vi "RampVoltagewithDDSv8.vi"() -> ()   [LabVIEW 2016]
uses:
  <vilib>/DAQmx/write.llb/DAQmx Write (Digital 1D Wfm NChan NSamp).vi
  <vilib>/DAQmx/write.llb/DAQmx Write (Analog 2D DBL NChan NSamp).vi
  <vilib>/DAQmx/create/channels.llb/DAQmx Create Channel (AO-Voltage-Basic).vi
  <vilib>/DAQmx/create/channels.llb/DAQmx Create Channel (DO-Digital Output).vi
  <vilib>/DAQmx/configure/timing.llb/DAQmx Timing (Sample Clock).vi
  <vilib>/DAQmx/configure/trigger.llb/DAQmx Start Trigger (Digital Edge).vi
  <vilib>/DAQmx/miscellaneous.llb/DAQmx Fill In Error Info.vi
  <vilib>/Waveform/DWDTOps.llb/DWDT Boolean Array to Digital.vi
  <vilib>/Waveform/DWDTOps.llb/DWDT Uncompress Digital.vi
  <vilib>/Waveform/DTblOps.llb/DTbl Digital to Analog.vi
  <resource>/objmgr/daqmx.rc
panel:
  in  "Reset P0.1":bool
  in  "Reset P0.0":bool
  in  "DDS Trigger delay (ms)":dbl step=0.01
  in  "DDS Trigger (Port 0 Line 1)":tag="Dev2/port0/line1"
  out "Digital Output":cluster{i32, dbl, dbl[][]}(graph)={0, 1e-05, [[5.0, 5.0, 5.0, 5.0, 5.0, 5.0, 5.0, 5.0, 5.0, 5.0, 5.0, 5.0, 5.0, 5.0, 5.0, 5.0, 5.0, 5.0, 5.0, 5.0, 5.0, 5.0, 5.0, 5.0, 5.0, 5.0, 5.0, 5.0, 5.0, 5.0, 5.0, 5.0, 5.0, 5.0, 5.0, 5.0, 5.0, 5.0, 5.0, 5.0, 5.0, 5.0, 5.0, 5.0, 5.0, 5.0, 5.0, 5.0, 5.0, 5.0, 5.0, 5.0, 5.0, 5.0, 5.0, 5.0, 5.0, 5.0, 5.0, 5.0, 5.0, 5.0, 5.0, 5.0, 5.0, 5.0, 5.0, 5.0, 5.0, 5.0, 5.0, 5.0, 5.0, 5.0, 5.0, 5.0, 5.0, 5.0, 5.0, 5.0, 5.0, 5.0, 5.0, 5.0, 5.0, 5.0, 5.0, 5.0, 5.0, 5.0, 5.0, 5.0, 5.0, 5.0, 5.0, 5.0, 5.0, 5.0, 5.0, 5.0, 0.0, 0.0, 0.0, 0.0, 0.0, 0.0, 0.0, 0.0, 0.0, 0.0, 0.0, 0.0, 0.0, 0.0, 0.0, 0.0, 0.0, 0.0, 0.0, 0.0, 0.0, 0.0, 0.0, 0.0, 0.0, 0.0, 0.0, 0.0, 0.0, 0.0, 0.0, 0.0, 0.0, 0.0, 0.0, 0.0, 0.0, 0.0, 0.0, 0.0, 0.0, 0.0, 0.0, 0.0, 0.0, 0.0, 0.0, 0.0, 0.0, 0.0, 0.0, 0.0, 0.0, 0.0, 0.0, 0.0, 0.0, 0.0, 0.0, 0.0, 0.0, 0.0, 0.0, 0.0, 0.0, 0.0, 0.0, 0.0, 0.0, 0.0, 0.0, 0.0, 0.0, 0.0, 0.0, 0.0, 0.0, 0.0, 0.0, 0.0, 0.0, 0.0, 0.0, 0.0, 0.0, 0.0, 0.0, 0.0, 0.0, 0.0, 0.0, 0.0, 0.0, 0.0, 0.0, 0.0, 0.0, 0.0, 0.0, 0.0, 0.0, 0.0, 0.0, 0.0, 0.0, 0.0, 0.0, 0.0, 0.0, 0.0, 0.0, 0.0, 0.0, 0.0, 0.0, 0.0, 0.0, 0.0, 0.0, 0.0, 0.0, 0.0, 0.0, 0.0, 0.0, 0.0, 0.0, 0.0, 0.0, 0.0, 0.0, 0.0, 0.0, 0.0, 0.0, 0.0, 0.0, 0.0, 0.0, 0.0, 0.0, 0.0, 0.0, 0.0, 0.0, 0.0, 0.0, 0.0, 0.0, 0.0, 0.0, 0.0, 0.0, 0.0, 0.0, 0.0, 0.0, 0.0, 0.0, 0.0, 0.0, 0.0, 0.0, 0.0, 0.0, 0.0, 0.0, 0.0, 0.0, 0.0, 0.0, 0.0, 0.0, 0.0, 0.0, 0.0, 0.0, 0.0, 0.0, 0.0, 0.0, 0.0, 0.0, 0.0, 0.0, 0.0, 0.0, 0.0, 0.0, 0.0, 0.0, 0.0, 0.0, 0.0, 0.0, 0.0, 0.0, 0.0, 0.0, 0.0, 5.0, 5.0, 5.0, 5.0, 5.0, 5.0, 5.0, 5.0, 5.0, 5.0, 5.0, 5.0, 5.0, 5.0, 5.0, 5.0, 5.0, 5.0, 5.0, 5.0, 5.0, 5.0, 5.0, 5.0, 5.0, 5.0, 5.0, 5.0, 5.0, 5.0, 5.0, 5.0, 5.0, 5.0, 5.0, 5.0, 5.0, 5.0, 5.0, 5.0, 5.0, 5.0, 5.0, 5.0, 5.0, 5.0, 5.0, 5.0, 5.0, 5.0, 5.0, 5.0, 5.0, 5.0, 5.0, 5.0, 5.0, 5.0, 5.0, 5.0, 5.0, 5.0, 5.0, 5.0, 5.0, 5.0, 5.0, 5.0, 5.0, 5.0, 5.0, 5.0, 5.0, 5.0, 5.0, 5.0, 5.0, 5.0, 5.0, 5.0, 5.0, 5.0, 5.0, 5.0, 5.0, 5.0, 5.0, 5.0, 5.0, 5.0, 5.0, 5.0, 5.0, 5.0, 5.0, 5.0, 5.0, 5.0, 5.0, 5.0, 5.0, 5.0, 5.0, 5.0, 5.0, 5.0, 5.0, 5.0, 5.0, 5.0, 5.0, 5.0, 5.0, 5.0, 5.0, 5.0, 5.0, 5.0, 5.0, 5.0, 5.0, 5.0, 5.0, 5.0, 5.0, 5.0, 5.0, 5.0, 5.0, 5.0, 5.0, 5.0, 5.0, 5.0, 5.0, 5.0, 5.0, 5.0, 5.0, 5.0, 5.0, 5.0, 5.0, 5.0, 5.0, 5.0, 5.0, 5.0, 5.0, 5.0, 5.0, 5.0, 5.0, 5.0, 5.0, 5.0, 5.0, 5.0, 5.0, 5.0, 5.0, 5.0, 5.0, 5.0, 5.0, 5.0, 5.0, 5.0, 5.0, 5.0, 5.0, 5.0, 5.0, 5.0, 5.0, 5.0, 5.0, 5.0, 5.0, 5.0, 5.0, 5.0, 5.0, 5.0, 5.0, 5.0, 5.0, 5.0, 5.0, 5.0, 5.0, 5.0, 5.0, 5.0, 5.0, 5.0, 5.0, 5.0, 5.0, 5.0, 0.0, 0.0, 0.0, 0.0, 0.0, 0.0, 0.0, 0.0, 0.0, 0.0, 0.0, 0.0, 0.0, 0.0, 0.0, 0.0, 0.0, 0.0, 0.0, 0.0, 0.0, 0.0, 0.0, 0.0, 0.0, 0.0, 0.0, 0.0, 0.0, 0.0, 0.0, 0.0, 0.0, 0.0, 0.0, 0.0, 0.0, 0.0, 0.0, 0.0, 0.0, 0.0, 0.0, 0.0, 0.0, 0.0, 0.0, 0.0, 0.0, 0.0, 0.0, 0.0, 0.0, 0.0, 0.0, 0.0, 0.0, 0.0, 0.0, 0.0, 0.0, 0.0, 0.0, 0.0, 0.0, 0.0, 0.0, 0.0, 0.0, 0.0, 0.0, 0.0, 0.0, 0.0, 0.0, 0.0, 0.0, 0.0, 0.0, 0.0, 0.0, 0.0, 0.0, 0.0, 0.0, 0.0, 0.0, 0.0, 0.0, 0.0, 0.0, 0.0, 0.0, 0.0, 0.0, 0.0, 0.0, 0.0, 0.0, 0.0, 0.0, 0.0, 0.0, 0.0, 0.0, 0.0, 0.0, 0.0, 0.0, 0.0, 0.0, 0.0, 0.0, 0.0, 0.0, 0.0, 0.0, 0.0, 0.0, 0.0, 0.0, 0.0, 0.0, 0.0, 0.0, 0.0, 0.0, 0.0, 0.0, 0.0, 0.0, 0.0, 0.0, 0.0, 0.0, 0.0, 0.0, 0.0, 0.0, 0.0, 0.0, 0.0, 0.0, 0.0, 0.0, 0.0, 0.0, 0.0, 0.0, 0.0, 0.0, 0.0, 0.0, 0.0, 0.0, 0.0, 0.0, 0.0, 0.0, 0.0, 0.0, 0.0, 0.0, 0.0, 0.0, 0.0, 0.0, 0.0, 0.0, 0.0, 0.0, 0.0, 0.0, 0.0, 0.0, 0.0, 0.0, 0.0, 0.0, 0.0, 0.0, 0.0, 0.0, 0.0, 0.0, 0.0, 0.0, 0.0, 0.0, 0.0, 0.0, 0.0, 0.0, 0.0, 0.0, 0.0, 0.0, 0.0, 0.0, 0.0, 5.0, 5.0, 5.0, 5.0, 5.0, 5.0, 5.0, 5.0, 5.0, 5.0, 5.0, 5.0, 5.0, 5.0, 5.0, 5.0, 5.0, 5.0, 5.0, 5.0, 5.0, 5.0, 5.0, 5.0, 5.0, 5.0, 5.0, 5.0, 5.0, 5.0, 5.0, 5.0, 5.0, 5.0, 5.0, 5.0, 5.0, 5.0, 5.0, 5.0, 5.0, 5.0, 5.0, 5.0, 5.0, 5.0, 5.0, 5.0, 5.0, 5.0, 5.0, 5.0, 5.0, 5.0, 5.0, 5.0, 5.0, 5.0, 5.0, 5.0, 5.0, 5.0, 5.0, 5.0, 5.0, 5.0, 5.0, 5.0, 5.0, 5.0, 5.0, 5.0, 5.0, 5.0, 5.0, 5.0, 5.0, 5.0, 5.0, 5.0, 5.0, 5.0, 5.0, 5.0, 5.0, 5.0, 5.0, 5.0, 5.0, 5.0, 5.0, 5.0, 5.0, 5.0, 5.0, 5.0, 5.0, 5.0, 5.0, 5.0, 5.0], [5.0, 5.0, 5.0, 5.0, 5.0, 5.0, 5.0, 5.0, 5.0, 5.0, 5.0, 5.0, 5.0, 5.0, 5.0, 5.0, 5.0, 5.0, 5.0, 5.0, 5.0, 5.0, 5.0, 5.0, 5.0, 5.0, 5.0, 5.0, 5.0, 5.0, 5.0, 5.0, 5.0, 5.0, 5.0, 5.0, 5.0, 5.0, 5.0, 5.0, 5.0, 5.0, 5.0, 5.0, 5.0, 5.0, 5.0, 5.0, 5.0, 5.0, 5.0, 5.0, 5.0, 5.0, 5.0, 5.0, 5.0, 5.0, 5.0, 5.0, 5.0, 5.0, 5.0, 5.0, 5.0, 5.0, 5.0, 5.0, 5.0, 5.0, 5.0, 5.0, 5.0, 5.0, 5.0, 5.0, 5.0, 5.0, 5.0, 5.0, 5.0, 5.0, 5.0, 5.0, 5.0, 5.0, 5.0, 5.0, 5.0, 5.0, 5.0, 5.0, 5.0, 5.0, 5.0, 5.0, 5.0, 5.0, 5.0, 5.0, 0.0, 0.0, 0.0, 0.0, 0.0, 0.0, 0.0, 0.0, 0.0, 0.0, 0.0, 0.0, 0.0, 0.0, 0.0, 0.0, 0.0, 0.0, 0.0, 0.0, 0.0, 0.0, 0.0, 0.0, 0.0, 0.0, 0.0, 0.0, 0.0, 0.0, 0.0, 0.0, 0.0, 0.0, 0.0, 0.0, 0.0, 0.0, 0.0, 0.0, 0.0, 0.0, 0.0, 0.0, 0.0, 0.0, 0.0, 0.0, 0.0, 0.0, 0.0, 0.0, 0.0, 0.0, 0.0, 0.0, 0.0, 0.0, 0.0, 0.0, 0.0, 0.0, 0.0, 0.0, 0.0, 0.0, 0.0, 0.0, 0.0, 0.0, 0.0, 0.0, 0.0, 0.0, 0.0, 0.0, 0.0, 0.0, 0.0, 0.0, 0.0, 0.0, 0.0, 0.0, 0.0, 0.0, 0.0, 0.0, 0.0, 0.0, 0.0, 0.0, 0.0, 0.0, 0.0, 0.0, 0.0, 0.0, 0.0, 0.0, 0.0, 0.0, 0.0, 0.0, 0.0, 0.0, 0.0, 0.0, 0.0, 0.0, 0.0, 0.0, 0.0, 0.0, 0.0, 0.0, 0.0, 0.0, 0.0, 0.0, 0.0, 0.0, 0.0, 0.0, 0.0, 0.0, 0.0, 0.0, 0.0, 0.0, 0.0, 0.0, 0.0, 0.0, 0.0, 0.0, 0.0, 0.0, 0.0, 0.0, 0.0, 0.0, 0.0, 0.0, 0.0, 0.0, 0.0, 0.0, 0.0, 0.0, 0.0, 0.0, 0.0, 0.0, 0.0, 0.0, 0.0, 0.0, 0.0, 0.0, 0.0, 0.0, 0.0, 0.0, 0.0, 0.0, 0.0, 0.0, 0.0, 0.0, 0.0, 0.0, 0.0, 0.0, 0.0, 0.0, 0.0, 0.0, 0.0, 0.0, 0.0, 0.0, 0.0, 0.0, 0.0, 0.0, 0.0, 0.0, 0.0, 0.0, 0.0, 0.0, 0.0, 0.0, 0.0, 0.0, 0.0, 0.0, 0.0, 0.0, 0.0, 0.0, 0.0, 0.0, 0.0, 0.0, 0.0, 0.0, 0.0, 0.0, 0.0, 0.0, 0.0, 0.0, 0.0, 0.0, 0.0, 0.0, 0.0, 0.0, 0.0, 0.0, 0.0, 0.0, 0.0, 0.0, 0.0, 0.0, 0.0, 0.0, 0.0, 0.0, 0.0, 0.0, 0.0, 0.0, 0.0, 0.0, 0.0, 0.0, 0.0, 0.0, 0.0, 0.0, 0.0, 0.0, 0.0, 0.0, 0.0, 0.0, 0.0, 0.0, 0.0, 0.0, 0.0, 0.0, 0.0, 0.0, 0.0, 0.0, 0.0, 0.0, 0.0, 0.0, 0.0, 0.0, 0.0, 0.0, 0.0, 0.0, 0.0, 0.0, 0.0, 0.0, 0.0, 0.0, 0.0, 0.0, 0.0, 0.0, 0.0, 0.0, 0.0, 0.0, 0.0, 0.0, 0.0, 0.0, 0.0, 0.0, 0.0, 0.0, 0.0, 0.0, 0.0, 0.0, 0.0, 0.0, 0.0, 0.0, 0.0, 0.0, 0.0, 0.0, 0.0, 0.0, 0.0, 0.0, 0.0, 0.0, 0.0, 0.0, 0.0, 0.0, 0.0, 0.0, 0.0, 0.0, 0.0, 0.0, 0.0, 0.0, 0.0, 0.0, 0.0, 0.0, 0.0, 0.0, 0.0, 0.0, 0.0, 0.0, 0.0, 0.0, 0.0, 0.0, 0.0, 0.0, 0.0, 0.0, 0.0, 0.0, 0.0, 0.0, 0.0, 0.0, 0.0, 0.0, 0.0, 0.0, 0.0, 0.0, 0.0, 0.0, 0.0, 0.0, 0.0, 0.0, 0.0, 0.0, 0.0, 0.0, 0.0, 0.0, 0.0, 0.0, 0.0, 0.0, 0.0, 0.0, 0.0, 0.0, 0.0, 0.0, 0.0, 0.0, 0.0, 0.0, 0.0, 0.0, 0.0, 0.0, 0.0, 0.0, 0.0, 0.0, 0.0, 0.0, 0.0, 0.0, 0.0, 0.0, 0.0, 0.0, 0.0, 0.0, 0.0, 0.0, 0.0, 0.0, 0.0, 0.0, 0.0, 0.0, 0.0, 0.0, 0.0, 0.0, 0.0, 0.0, 0.0, 0.0, 0.0, 0.0, 0.0, 0.0, 0.0, 0.0, 0.0, 0.0, 0.0, 0.0, 0.0, 0.0, 0.0, 0.0, 0.0, 0.0, 0.0, 0.0, 0.0, 0.0, 0.0, 0.0, 0.0, 0.0, 0.0, 0.0, 0.0, 0.0, 0.0, 0.0, 0.0, 0.0, 0.0, 0.0, 0.0, 0.0, 0.0, 0.0, 0.0, 0.0, 0.0, 0.0, 0.0, 0.0, 0.0, 0.0, 0.0, 0.0, 0.0, 0.0, 0.0, 0.0, 0.0, 0.0, 0.0, 0.0, 0.0, 0.0, 0.0, 0.0, 0.0, 0.0, 0.0, 0.0, 0.0, 0.0, 0.0, 0.0, 0.0, 0.0, 0.0, 0.0, 0.0, 0.0, 0.0, 0.0, 0.0, 0.0, 0.0, 0.0, 0.0, 0.0, 0.0, 0.0, 0.0, 0.0, 0.0, 0.0, 0.0, 0.0, 0.0, 0.0, 0.0, 0.0, 0.0, 0.0, 0.0, 0.0, 0.0, 0.0, 0.0, 0.0, 0.0, 0.0, 0.0, 0.0, 0.0, 0.0, 0.0, 0.0, 0.0, 0.0, 0.0, 0.0, 0.0, 0.0, 0.0, 0.0, 0.0, 0.0, 0.0, 0.0, 0.0, 0.0, 0.0, 0.0, 0.0, 0.0, 0.0, 0.0, 0.0, 0.0, 0.0, 0.0, 0.0, 0.0, 0.0, 0.0, 0.0, 0.0, 0.0, 0.0, 0.0, 0.0, 0.0, 0.0, 0.0, 0.0, 0.0, 0.0, 0.0, 0.0, 0.0, 0.0, 0.0, 0.0, 0.0, 0.0, 0.0, 0.0, 0.0, 0.0, 0.0, 0.0, 0.0, 0.0, 0.0, 0.0, 0.0, 0.0, 0.0, 0.0, 0.0, 0.0, 0.0, 0.0, 0.0, 0.0, 0.0, 0.0, 0.0, 0.0, 0.0, 0.0, 0.0, 0.0, 0.0, 0.0, 0.0, 0.0, 0.0, 0.0, 0.0, 0.0, 0.0, 0.0, 0.0, 0.0, 0.0, 0.0, 0.0, 0.0, 0.0, 0.0, 0.0, 0.0, 0.0, 0.0, 0.0, 0.0, 0.0, 0.0, 0.0, 0.0, 0.0, 0.0, 0.0, 0.0, 0.0, 0.0, 0.0, 0.0, 0.0, 0.0, 0.0, 0.0, 0.0, 0.0, 0.0, 0.0, 0.0, 0.0, 0.0, 0.0, 0.0, 0.0, 0.0, 0.0, 0.0, 0.0, 0.0, 0.0, 0.0, 0.0, 0.0, 0.0, 0.0, 0.0, 0.0, 0.0, 0.0, 0.0, 0.0, 0.0, 0.0, 0.0, 0.0, 0.0, 0.0, 0.0, 0.0, 0.0, 0.0, 0.0, 0.0, 0.0, 0.0, 0.0, 0.0, 0.0, 0.0, 0.0, 0.0, 0.0, 0.0, 0.0, 0.0, 0.0, 0.0, 0.0, 0.0, 0.0, 0.0, 0.0, 0.0, 0.0, 0.0, 0.0, 5.0]]}
  out "Analog Outputs":cluster{i32, dbl, dbl[][]}(graph)={0, 4e-06, array4x2001[8004 elements]}
  in  "High Gain Switch (Port 0 Line 0)":tag="Dev2/port0/line0"
  in  "Ramp to high gain \ndelay (ms)":dbl step=0.01
  in  "error in 2":errorcluster caption="error in"
  in  "ao3 ramp amplitude (V)":dbl=0.4
  in  "ao2 ramp amplitude (V)":dbl=0.3
  in  "ao1 ramp amplitude (V)":dbl=0.2
  in  "SolsTiS 2 - Fast Piezo (ao3)":tag="Dev2/ao3"
  in  "SolsTiS 2 - Slow Piezo (ao2)":tag="Dev2/ao2"
  out "size(s)":i32=2001
  in  "Trigger delay NI (ms)":dbl=1.0
  in  "Trigger Input (PFI0)":tag="/Dev2/PFI0"
  in  "SolsTiS 1 - Fast Piezo (ao1)":tag="Dev2/ao1"
  in  "SolsTiS 1 - Slow Piezo (ao0)":tag="Dev2/ao0"
  in  "Plateau duration (ms)":dbl=2.0 step=0.01
  in  "Ramp duration (ms)":dbl=2.0 step=0.01
  in  "ao0 ramp amplitude (V)":dbl=1.0 step=0.001
  in  "error in":errorcluster
  # "MAGIS LASER SYSTEM\nChirp Control"
  # "Ramp Definition"
  # "Output Monitor"
  # "Channel Definition"
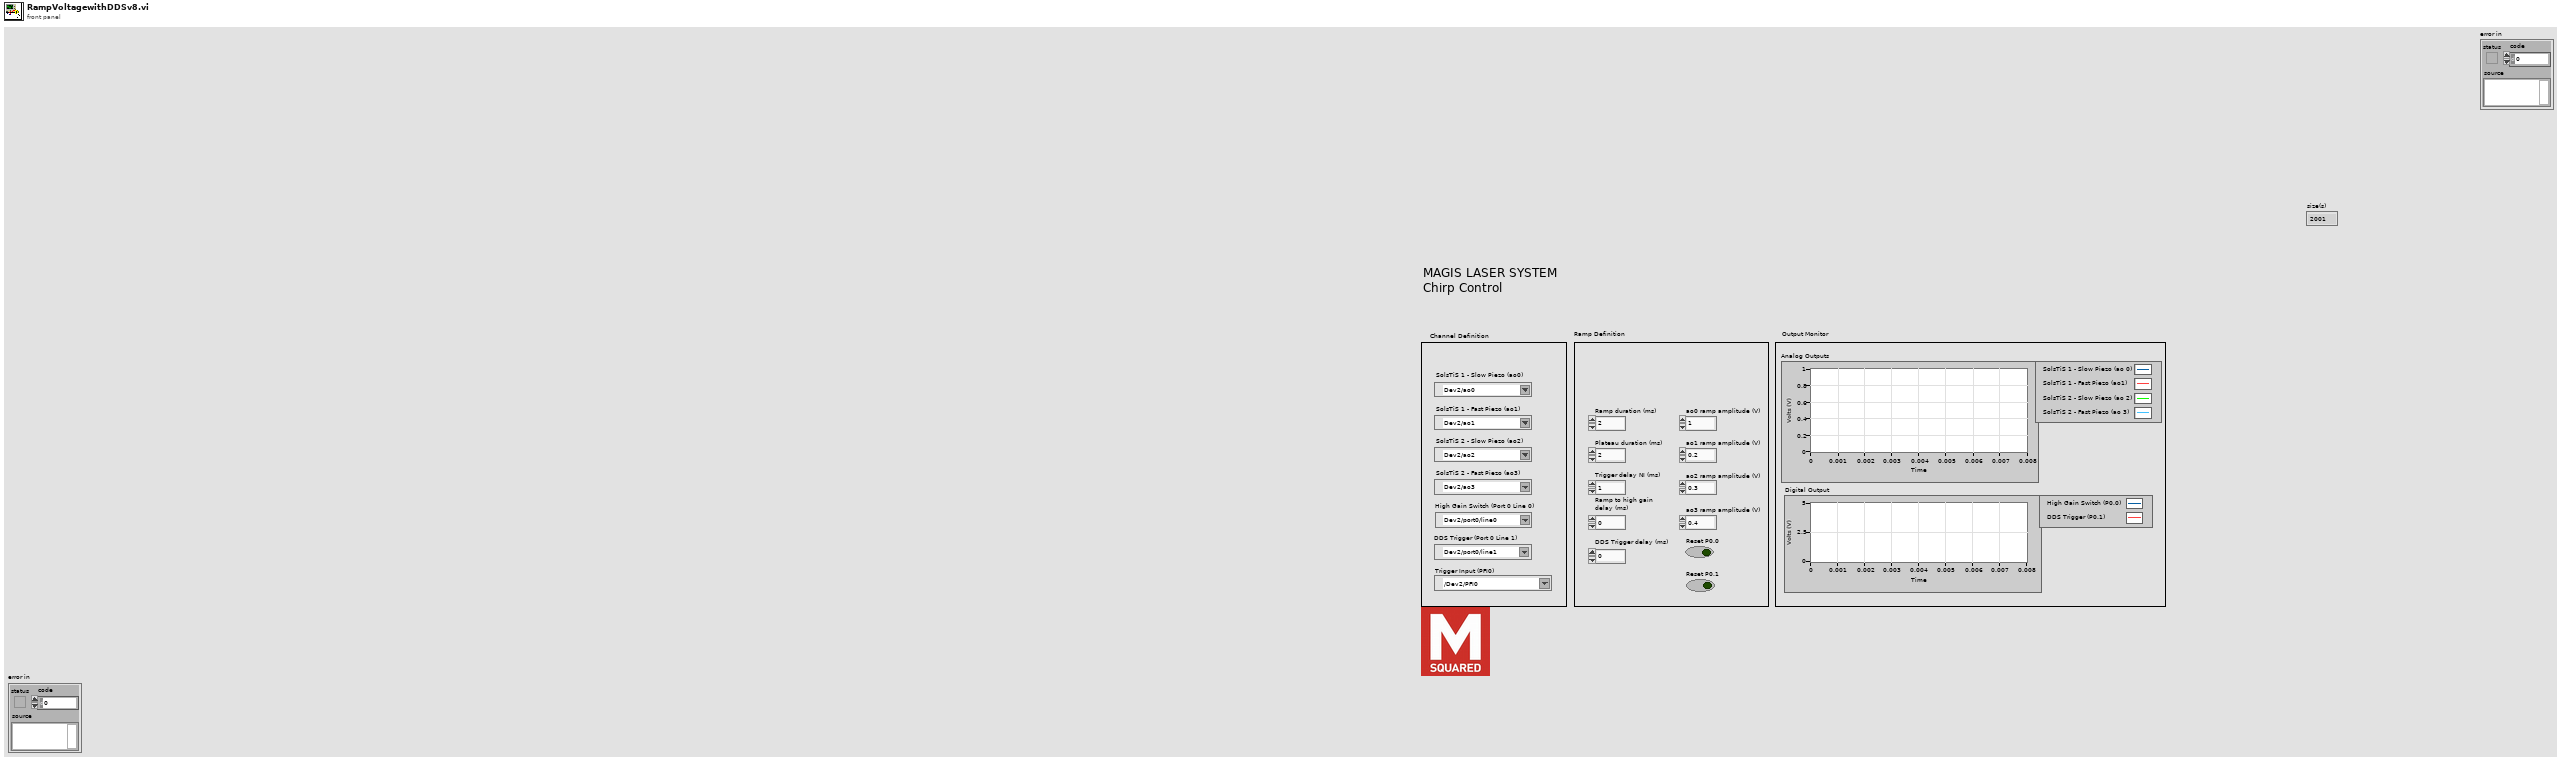
[diagram p1: front panel]
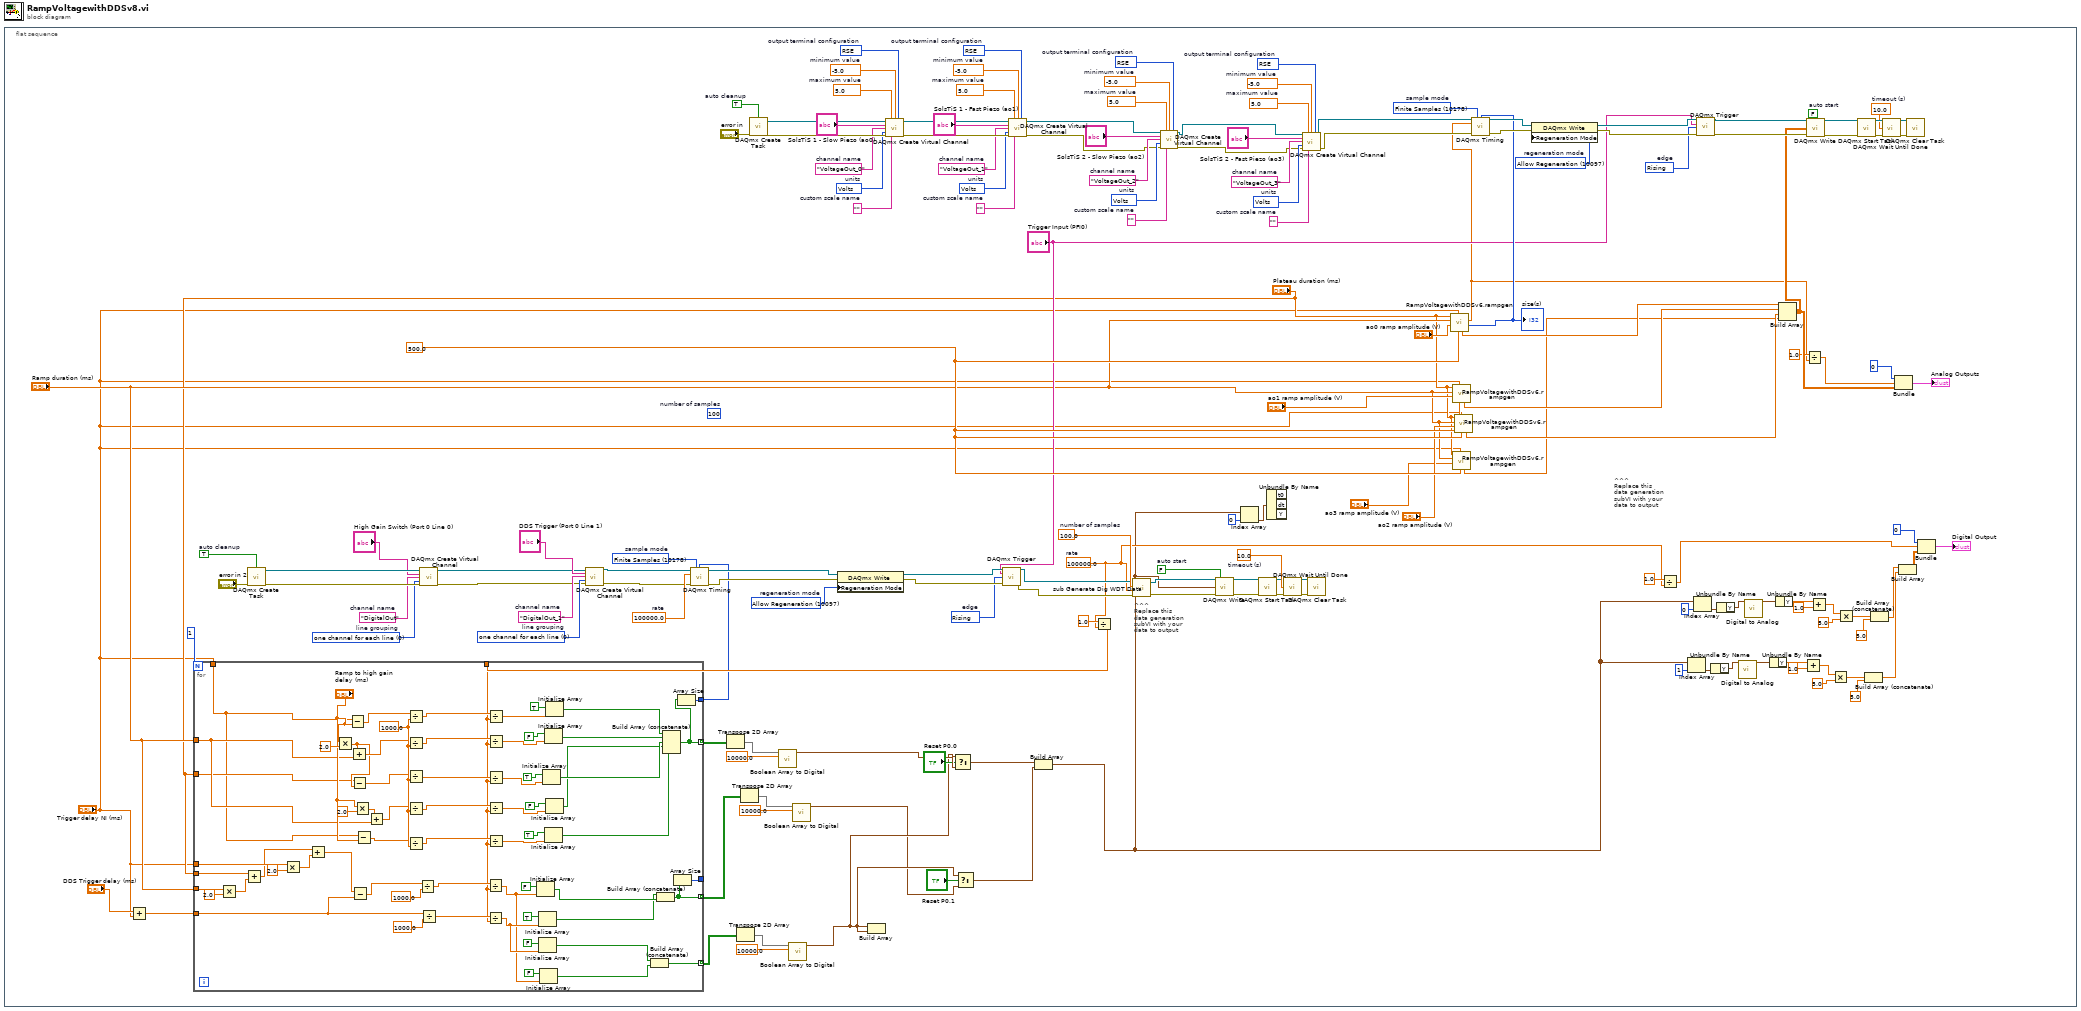
[diagram p0: block diagram]
diagram:
  n1 = flat-sequence {
    frame #0 {
      w37 = 0 items=["one channel for each line", "one channel for all lines"]  # line grouping
      w36 = "DigitalOut_1"  # channel name
      w105 = 500.0 ("No of samples in ramp (500 or less)")
      w72 = 10280 items=["Rising"=10280, "Falling"=10171]  # edge
      w74 = 10097 items=["Allow Regeneration"=10097, "Do Not Allow Regeneration"=10158]  # regeneration mode
      w77 = 10178 items=["Finite Samples"=10178, "Continuous Samples"=10123, "Hardware Timed Single Point"=12522]  # sample mode
      (unwired) 100  # number of samples
      w78 = 100000.0  # rate
      w81 = 0 items=["one channel for each line", "one channel for all lines"]  # line grouping
      w80 = "DigitalOut"  # channel name
      w83 = TRUE  # auto cleanup
      w98 = 10.0  # timeout (s)
      w46 = 100000.0  # rate
      w91 = 100.0  # number of samples
      w88 = FALSE  # auto start
      w112 = 10083 items=["Default"=-1, "RSE"=10083, "Differential"=10106, "Pseudodifferential"=12529]  # output terminal configuration
      w113 = 10348 items=["Volts"=10348, "From Custom Scale"=10065]  # units
      w114 = "VoltageOut_3"  # channel name
      w115 = ""  # custom scale name
      w116 = -5.0  # minimum value
      w117 = 5.0  # maximum value
      w121 = 10083 items=["Default"=-1, "RSE"=10083, "Differential"=10106, "Pseudodifferential"=12529]  # output terminal configuration
      w122 = 10348 items=["Volts"=10348, "From Custom Scale"=10065]  # units
      w123 = "VoltageOut_2"  # channel name
      w124 = ""  # custom scale name
      w125 = -5.0  # minimum value
      w126 = 5.0  # maximum value
      w133 = 10280 items=["Rising"=10280, "Falling"=10171]  # edge
      w135 = 10097 items=["Allow Regeneration"=10097, "Do Not Allow Regeneration"=10158]  # regeneration mode
      w138 = 10178 items=["Finite Samples"=10178, "Continuous Samples"=10123, "Hardware Timed Single Point"=12522]  # sample mode
      w140 = 10083 items=["Default"=-1, "RSE"=10083, "Differential"=10106, "Pseudodifferential"=12529]  # output terminal configuration
      w141 = 10348 items=["Volts"=10348, "From Custom Scale"=10065]  # units
      w142 = "VoltageOut_1"  # channel name
      w143 = ""  # custom scale name
      w144 = -5.0  # minimum value
      w145 = 5.0  # maximum value
      w147 = 10083 items=["Default"=-1, "RSE"=10083, "Differential"=10106, "Pseudodifferential"=12529]  # output terminal configuration
      w148 = 10348 items=["Volts"=10348, "From Custom Scale"=10065]  # units
      w149 = "VoltageOut_0"  # channel name
      w151 = ""  # custom scale name
      w152 = -5.0  # minimum value
      w153 = 5.0  # maximum value
      w155 = TRUE  # auto cleanup
      w161 = 10.0  # timeout (s)
      w165 = FALSE  # auto start
      # "^^^\nReplace this\ndata generation\nsubVI with your\ndata to output"
      # "^^^\nReplace this\ndata generation\nsubVI with your\ndata to output"
      n2 = Add(x="DDS Trigger delay (ms)", y="Trigger delay NI (ms)") -> (x+y=w29:dbl)
      n3 = call <vilib>:"DAQmx Create Task.vi"("auto cleanup"=w83, "error in"="error in 2") -> ("task out"=w82:refnum<k21>, "error out"=w84:errorcluster)  [unwired: 12 in]
      n4 = call-poly <vilib>:"DAQmx Create Virtual Channel.vi"("task in"=w82, "lines"="High Gain Switch (Port 0 Line 0)", "name to assign"=w80, "line grouping"=w81, "error in"=w84) -> ("task out"=w31:refnum<k21>, "error out"=w34:errorcluster)  [unwired: 9 in]
      n5 = call-poly <vilib>:"DAQmx Create Virtual Channel.vi"("task in"=w31, "lines"="DDS Trigger (Port 0 Line 1)", "name to assign"=w36, "line grouping"=w37, "error in"=w34) -> ("task out"=w33:refnum<k21>, "error out"=w32:errorcluster)  [unwired: 9 in]
      n6 = call <vilib>:"DAQmx Create Task.vi"("auto cleanup"=w155, "error in"="error in") -> ("task out"=w154:refnum<k21>, "error out"=w156:errorcluster)  [unwired: 12 in]
      n7 = call-poly <vilib>:"DAQmx Create Virtual Channel.vi"("task in"=w154, "maximum value"=w153, "minimum value"=w152, "output terminal configuration"=w147, "physical channels"="SolsTiS 1 - Slow Piezo (ao0)", "name to assign"=w149, "units"=w148, "error in"=w156, "custom scale name"=w151) -> ("task out"=w146:refnum<k21>, "error out"=w150:errorcluster)  [unwired: 5 in]
      n8 = call-poly <vilib>:"DAQmx Create Virtual Channel.vi"("task in"=w146, "maximum value"=w145, "minimum value"=w144, "output terminal configuration"=w140, "physical channels"="SolsTiS 1 - Fast Piezo (ao1)", "name to assign"=w142, "units"=w141, "error in"=w150, "custom scale name"=w143) -> ("task out"=w119:refnum<k21>, "error out"=w118:errorcluster)  [unwired: 5 in]
      n9 = Divide(x=1.0, y=w46) -> (x/y=w68:dbl)
      n10 = for {
        N: 1 -> [_]
        tunnel: w68 -> [w182]
        tunnel: [w209] -> w65 mode=indexing
        tunnel: [w208] -> w64
        tunnel: "Ramp duration (ms)" -> [w197]
        tunnel: "Plateau duration (ms)" -> [w196]
        tunnel: "Trigger delay NI (ms)" -> [w195]
        tunnel: w29 -> [w188]
        tunnel: "Ramp duration (ms)" -> [w192]
        tunnel: "Plateau duration (ms)" -> [w189]
        tunnel: [w179] -> _
        tunnel: "Trigger delay NI (ms)" -> [w176]
        tunnel: [w173] -> w23 mode=indexing
        tunnel: [w166] -> w20 mode=indexing
        w228 = 1000.0
        n11 = Multiply(x=w192, y=2.0) -> (x*y=w190:dbl)
        n12 = Add(x=w189, y=w190) -> (x+y=w175:dbl)
        n13 = Multiply(x=w176, y=2.0) -> (x*y=w177:dbl)
        n14 = Add(x=w175, y=w177) -> (x+y=w174:dbl)
        n15 = Multiply(x="Ramp to high gain \ndelay (ms)", y=2.0) -> (x*y=w204:dbl)
        n16 = Subtract(x=w195, y="Ramp to high gain \ndelay (ms)") -> (x-y=w207:dbl)
        n17 = Add(x=w204, y=w197) -> (x+y=w205:dbl)
        n18 = Subtract(x=w196, y=w204) -> (x-y=w203:dbl)
        n19 = Subtract(x=w174, y=w188) -> (x-y=w185:dbl)
        n20 = Multiply(x="Ramp to high gain \ndelay (ms)", y=2.0) -> (x*y=w201:dbl)
        n21 = Subtract(x=w195, y="Ramp to high gain \ndelay (ms)") -> (x-y=w198:dbl)
        n22 = Add(x=w201, y=w197) -> (x+y=w200:dbl)
        n23 = Divide(x=w207, y=w228) -> (x/y=w227:dbl)
        n24 = Divide(x=w205, y=w228) -> (x/y=w226:dbl)
        n25 = Divide(x=w203, y=w228) -> (x/y=w225:dbl)
        n26 = Divide(x=w200, y=w228) -> (x/y=w224:dbl)
        n27 = Divide(x=w198, y=w228) -> (x/y=w223:dbl)
        n28 = Divide(x=w185, y=1000.0) -> (x/y=w184:dbl)
        n29 = Divide(x=w188, y=1000.0) -> (x/y=w183:dbl)
        n30 = Divide(x=w184, y=w182) -> (x/y=w169:dbl)
        n31 = Divide(x=w183, y=w182) -> (x/y=w170:dbl)
        n32 = Divide(x=w227, y=w182) -> (x/y=w219:dbl)
        n33 = Divide(x=w226, y=w182) -> (x/y=w218:dbl)
        n34 = Divide(x=w225, y=w182) -> (x/y=w217:dbl)
        n35 = Divide(x=w224, y=w182) -> (x/y=w216:dbl)
        n36 = Divide(x=w223, y=w182) -> (x/y=w215:dbl)
        n37 = Initialize Array(FALSE, w169) -> (w181:bool[])
        n38 = Initialize Array(TRUE, w170) -> (w180:bool[])
        n39 = Initialize Array(FALSE, w170) -> (w168:bool[])
        n40 = Initialize Array(FALSE, w169) -> (w167:bool[])
        n41 = Initialize Array(TRUE, w217) -> (w212:bool[])
        n42 = Initialize Array(FALSE, w218) -> (w213:bool[])
        n43 = Initialize Array(TRUE, w215) -> (w210:bool[])
        n44 = Initialize Array(TRUE, w219) -> (w214:bool[])
        n45 = Initialize Array(FALSE, w216) -> (w211:bool[])
        n46 = Build Array (concatenate)(w168, w167) -> (w166:bool[])
        n47 = Build Array (concatenate)(w180, w181) -> (w173:bool[])
        n48 = Build Array (concatenate)(w214, w213, w212, w211, w210) -> (w209:bool[])
        n49 = Array Size(array=w173) -> (size(s)=w179:i32)
        n50 = Array Size(array=w209) -> (size(s)=w208:i32)
      }
      n51 = call-poly <vilib>:"DAQmx Timing.vi"("task/channels in"=w33, "sample mode"=w77, "samples per channel"=w64, "rate"=w78, "error in"=w32) -> ("task out"=w76:refnum<k21>, "error out"=w79:errorcluster)  [unwired: 9 in]
      n52 = Transpose 2D Array(2D array=w65) -> (transposed array=w66:bool[][])
      n53 = Transpose 2D Array(2D array=w20) -> (transposed array=w21:bool[][])
      n54 = Transpose 2D Array(2D array=w23) -> (transposed array=w24:bool[][])
      n55 = call-poly <vilib>:"Boolean Array to Digital.vi"("sample rate"=10000.0, "boolean array"=w66) -> ("digital waveform"=w8:digitalwaveform)  [unwired: 8 in, 1 out]
      n56 = call-poly <vilib>:"Boolean Array to Digital.vi"("sample rate"=10000.0, "boolean array"=w21) -> ("digital waveform"=w5:digitalwaveform)  [unwired: 8 in, 1 out]
      n57 = call-poly <vilib>:"Boolean Array to Digital.vi"("sample rate"=10000.0, "boolean array"=w24) -> ("digital waveform"=w4:digitalwaveform)  [unwired: 8 in, 1 out]
      n58 = property class="DAQmx Write"(reference=w76, error in=w79, "Regeneration Mode"=w74) -> (reference out=w73:refnum<k21>, error out=w75:errorcluster)
      n59 = Build Array(w5, w5) -> ()  [unwired: 1 out]
      n60 = Select(t=w5, s="Reset P0.0", f=w8) -> (s? t:f=w3:digitalwaveform)
      n61 = Select(t=w5, s="Reset P0.1", f=w4) -> (s? t:f=w2:digitalwaveform)
      n62 = call-poly <vilib>:"DAQmx Trigger.vi"("task/channels in"=w73, "source"="Trigger Input (PFI0)", "edge"=w72, "error in"=w75) -> ("task out"=w71:refnum<k21>, "error out"=w70:errorcluster)  [unwired: 10 in]
      n63 = Build Array(w3, w2) -> (w1:digitalwaveform[])
      n64 = call <vilib>:"sub Generate Dig WDT Data.vi"("task in"=w71, "number of samples"=w91, "update rate"=w46, "error in"=w70) -> ("task out"=w90:refnum<k21>, "error out"=w89:errorcluster)  [unwired: 1 in, 1 out]
      n65 = call-poly <vilib>:"DAQmx Create Virtual Channel.vi"("task in"=w119, "maximum value"=w126, "minimum value"=w125, "output terminal configuration"=w121, "physical channels"="SolsTiS 2 - Slow Piezo (ao2)", "name to assign"=w123, "units"=w122, "error in"=w118, "custom scale name"=w124) -> ("task out"=w110:refnum<k21>, "error out"=w109:errorcluster)  [unwired: 5 in]
      n66 = call-poly <vilib>:"DAQmx Write.vi"("task/channels in"=w90, "auto start"=w88, "data"=w1, "error in"=w89) -> ("task out"=w95:refnum<k21>, "error out"=w96:errorcluster)  [unwired: 9 in, 1 out]
      n67 = Index Array(array=w1, index=0) -> (element=w86:digitalwaveform)
      n68 = call <vilib>:"DAQmx Start Task.vi"("task/channels in"=w95, "error in"=w96) -> ("task out"=w92:refnum<k21>, "error out"=w93:errorcluster)  [unwired: 12 in]
      n69 = Unbundle By Name(w86) -> ()  [unwired: 3 out]
      n70 = call <vilib>:"DAQmx Wait Until Done.vi"("task/channels in"=w92, "timeout (sec)"=w98, "error in"=w93) -> ("task out"=w97:refnum<k21>, "error out"=w94:errorcluster)  [unwired: 11 in]
      n71 = call-poly <vilib>:"DAQmx Create Virtual Channel.vi"("task in"=w110, "maximum value"=w117, "minimum value"=w116, "output terminal configuration"=w112, "physical channels"="SolsTiS 2 - Fast Piezo (ao3)", "name to assign"=w114, "units"=w113, "error in"=w109, "custom scale name"=w115) -> ("task out"=w107:refnum<k21>, "error out"=w108:errorcluster)  [unwired: 5 in]
      n72 = call <vilib>:"DAQmx Clear Task.vi"("task in"=w97, "error in"=w94) -> ()  [unwired: 13 in, 1 out]
      n73 = call "RampVoltagewithDDSv6,rampgen.vi"("No of samples in ramp"=w105, "Trigger delay NI (ms)"="Trigger delay NI (ms)", "Ramp Amplitude (V)}"="ao0 ramp amplitude (V)", "Ramp duration (ms)"="Ramp duration (ms)", "Plateau duration (ms)"="Plateau duration (ms)") -> ("Numeric 2"=w129:i32, "Numeric"=w49:dbl, "Array"=w106:dbl[])  [unwired: 3 in, 1 out]
      "size(s)" <- w129
      n74 = call "RampVoltagewithDDSv6,rampgen.vi"("No of samples in ramp"=w105, "Trigger delay NI (ms)"="Trigger delay NI (ms)", "Ramp Amplitude (V)}"="ao1 ramp amplitude (V)", "Ramp duration (ms)"="Ramp duration (ms)", "Plateau duration (ms)"="Plateau duration (ms)") -> ("Array"=w101:dbl[])  [unwired: 3 in, 3 out]
      n75 = call "RampVoltagewithDDSv6,rampgen.vi"("No of samples in ramp"=w105, "Trigger delay NI (ms)"="Trigger delay NI (ms)", "Ramp Amplitude (V)}"="ao3 ramp amplitude (V)", "Ramp duration (ms)"="Ramp duration (ms)", "Plateau duration (ms)"="Plateau duration (ms)") -> ("Array"=w99:dbl[])  [unwired: 3 in, 3 out]
      n76 = call "RampVoltagewithDDSv6,rampgen.vi"("No of samples in ramp"=w105, "Trigger delay NI (ms)"="Trigger delay NI (ms)", "Ramp Amplitude (V)}"="ao2 ramp amplitude (V)", "Ramp duration (ms)"="Ramp duration (ms)", "Plateau duration (ms)"="Plateau duration (ms)") -> ("Array"=w100:dbl[])  [unwired: 3 in, 3 out]
      n77 = call-poly <vilib>:"DAQmx Timing.vi"("task/channels in"=w107, "sample mode"=w138, "samples per channel"=w129, "rate"=w49, "error in"=w108) -> ("task out"=w137:refnum<k21>, "error out"=w139:errorcluster)  [unwired: 9 in]
      n78 = property class="DAQmx Write"(reference=w137, error in=w139, "Regeneration Mode"=w135) -> (reference out=w134:refnum<k21>, error out=w136:errorcluster)
      n79 = Divide(x=1.0, y=w46) -> (x/y=w45:dbl)
      n80 = Index Array(array=w1, index=1) -> (element=w18:digitalwaveform)
      n81 = Index Array(array=w1, index=0) -> (element=w56:digitalwaveform)
      n82 = call-poly <vilib>:"DAQmx Trigger.vi"("task/channels in"=w134, "source"="Trigger Input (PFI0)", "edge"=w133, "error in"=w136) -> ("task out"=w131:refnum<k21>, "error out"=w130:errorcluster)  [unwired: 10 in]
      n83 = Unbundle By Name(w18) -> ("Y"=w17:digitaldata)
      n84 = Unbundle By Name(w56) -> ("Y"=w55:digitaldata)
      n85 = call-poly <vilib>:"Digital to Analog.vi"("digital table"=w17) -> ("analog waveform"=w16:waveform(dbl))  [unwired: 7 in, 3 out]
      n86 = call-poly <vilib>:"Digital to Analog.vi"("digital table"=w55) -> ("analog waveform"=w54:waveform(dbl))  [unwired: 7 in, 3 out]
      n87 = Unbundle By Name(w16) -> ("Y"=w14:dbl[])
      n88 = Unbundle By Name(w54) -> ("Y"=w43:dbl[])
      n89 = Build Array(w106, w101, w100, w99) -> (w60:dbl[][])
      n90 = Add(x=w14, y=1.0) -> (x+y=w13:dbl[])
      n91 = Divide(x=1.0, y=w49) -> (x/y=w48:dbl)
      n92 = call-poly <vilib>:"DAQmx Write.vi"("task/channels in"=w131, "auto start"=w165, "data"=w60, "error in"=w130) -> ("task out"=w160:refnum<k21>, "error out"=w159:errorcluster)  [unwired: 9 in, 1 out]
      n93 = Add(x=w43, y=1.0) -> (x+y=w42:dbl[])
      n94 = Multiply(x=w13, y=5.0) -> (x*y=w11:dbl[])
      n95 = Multiply(x=w42, y=5.0) -> (x*y=w40:dbl[])
      n96 = call <vilib>:"DAQmx Start Task.vi"("task/channels in"=w160, "error in"=w159) -> ("task out"=w164:refnum<k21>, "error out"=w163:errorcluster)  [unwired: 12 in]
      n97 = Build Array (concatenate)(w11, 5.0 ("y")) -> (w9:dbl[])
      n98 = Build Array (concatenate)(w40, 5.0 ("y")) -> (w38:dbl[])
      n99 = call <vilib>:"DAQmx Wait Until Done.vi"("task/channels in"=w164, "timeout (sec)"=w161, "error in"=w163) -> ("task out"=w158:refnum<k21>, "error out"=w162:errorcluster)  [unwired: 11 in]
      n100 = Bundle(0, w48, w60) -> (→"Analog Outputs":cluster{i32, dbl, dbl[][]})  [unwired: 1 in]
      n101 = Build Array(w38, w9) -> (w51:dbl[][])
      n102 = call <vilib>:"DAQmx Clear Task.vi"("task in"=w158, "error in"=w162) -> ()  [unwired: 13 in, 1 out]
      n103 = Bundle(0, w45, w51) -> (→"Digital Output":cluster{i32, dbl, dbl[][]})  [unwired: 1 in]
    }
  }
